vi "Check for Devices Present.vi"(6 "stop notifier reference":refnum<notifier>, 8 "error in":errorcluster, 10 "Devices in":T1[](array[typedef]), 11 "Startup Optimization in":refnum<class "Startup Optimization.lvclass">) -> (0 "error out":errorcluster, 2 "Failed Devices":T1[](array[typedef]), 3 "Startup Optimization out":refnum<class "Startup Optimization.lvclass">, 4 "Time has Elapsed":bool)   [LabVIEW 2018, in "Startup Optimization Actor.lvlib" / "Startup Optimization.lvclass"]
doc: "Ensure all devices that have been told to activate have been activated."
uses:
  Startup Optimization.lvclass
  <vilib>/ORNL/CSEISMIC DDS/CSEISMIC DDS Base/Data Types/Controls/DeviceID.ctl
  C:/Users/Administrator/Desktop/2018LabVIEW EMS/EMS Generic Actor/EMS Generic/EMS Generic.lvclass
  EMS Generic Actor/EMS Generic/EMS Generic.lvclass
  <vilib>/ORNL/CSEISMIC DDS/CSEISMIC DDS Base/CSEISMIC DDS.lvclass
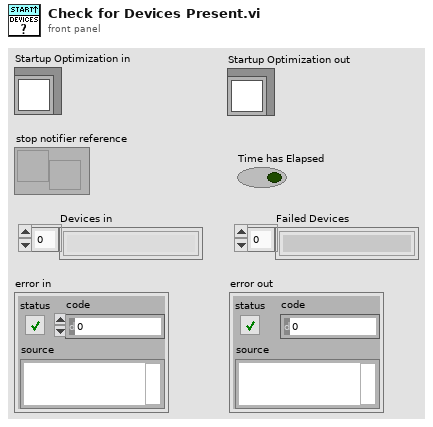
[diagram p1: front panel]
types:
  T1 = typedef "CSEISMIC DDS.lvlib/CSEISMIC DDS.lvclass/DeviceID.ctl" = string
  T2 = typedef "CSEISMIC DDS.lvlib/CSEISMIC DDS.lvclass/IED_Status.ctl" = cluster{"DeviceID":T1, "Timestamp":T3, "MicrogridID":u8, "Active":bool, "Inactive":bool, "Error":i32, "Fault":bool, "ErrorString":string}
  T3 = typedef "CSEISMIC DDS.lvlib/CSEISMIC DDS.lvclass/Timestamp.ctl" = cluster{"Seconds":u64, "Remainder":u64}
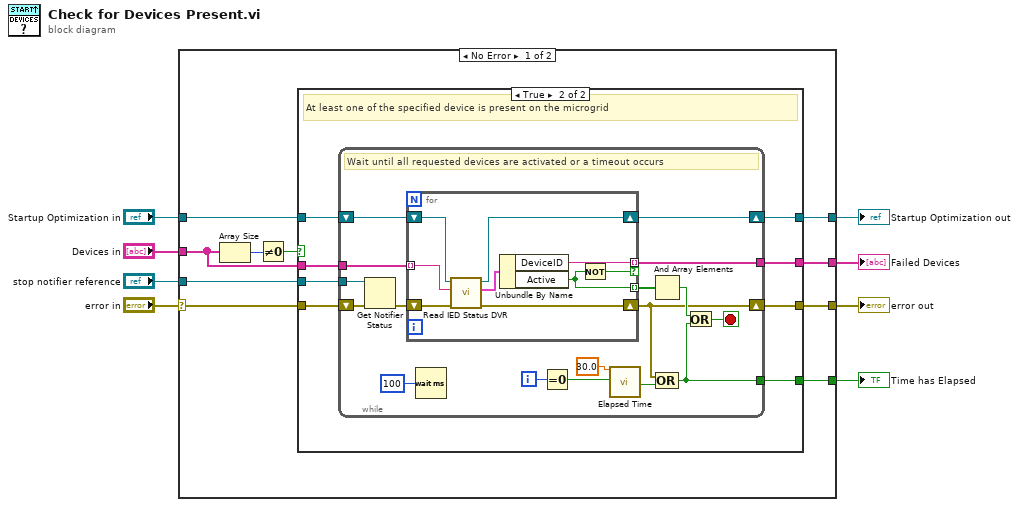
[diagram p0: block diagram]
diagram:
  n1 = case shown="No Error" "error in" {
    selector: "error in" -> [w14 w57]
    tunnel: [w18 w57] -> w8
    tunnel: [w17 w56] -> w7
    tunnel: "stop notifier reference" -> [w16 _]
    tunnel: [w15 _] -> w5
    tunnel: [w11 w55] -> w3
    tunnel: "Startup Optimization in" -> [w10 w55]
    tunnel: "Devices in" -> [w9 w56]
    frame No Error {
      n2 = Array Size(array=w9) -> (size(s)=w12:i32)
      n3 = Not Equal To 0?(x=w12) -> (x != 0?=w13:bool)
      n4 = case shown="True" w13 {
        tunnel: w10 -> [w19 w28]
        tunnel: w9 -> [_ w27]
        tunnel: w14 -> [w20 w26]
        tunnel: [_ w25] -> w15
        tunnel: w16 -> [_ w24]
        tunnel: [_ w23] -> w17
        tunnel: [w20 w22] -> w18
        tunnel: [w19 w21] -> w11
        frame False {
          # "No devices in the list are on the system.  Move to next type of device."
        }
        frame True {
          # "At least one of the specified device is present on the microgrid"
          n5 = while {
            tunnel: w27 -> [w44]
            tunnel: [w38] -> w25
            tunnel: w24 -> [w37]
            tunnel: [w33] -> w23
            shift-right: [w29] -> w22
            shift-left: w26 -> [w32]
            shift-right: [w31] -> w21
            shift-left: w28 -> [w45]
            i -> [w36]
            stop <- w40 stop-if-true
            # "Wait until all requested devices are activated or a timeout occurs"
            n6 = Get Notifier Status(notifier=w37, error in (no error)=w32) -> (error out=w30:errorcluster)  [unwired: 4 out]
            n7 = for {
              tunnel: w44 -> [w49] mode=indexing
              tunnel: [w53] -> w43 mode=indexing
              tunnel: [w54] -> w33 mode=indexing if=w52
              shift-right: [w50] -> w31
              shift-left: w45 -> [w51]
              shift-right: [w46] -> w29
              shift-left: w30 -> [w47]
              n8 = call "Read IED Status DVR.vi"("error in"=w47, "DeviceID"=w49, "EMS Generic in"=w51) -> ("error out"=w46:errorcluster, "IED_Status"=w48:T2, "EMS Generic out"=w50:refnum<class "Startup Optimization.lvclass">)  [unwired: 5 in, 1 out]
              n9 = Unbundle By Name(w48) -> ("DeviceID"=w54:T1, "Active"=w53:bool)
              n10 = Not(x=w53) -> (.not. x?=w52:bool)
            }
            n11 = Wait (ms)(milliseconds to wait=u32 100) -> ()  [unwired: 1 out]
            n12 = Equal To 0?(x=w36) -> (x = 0?=w35:bool)
            n13 = call "Elapsed Time"("Time Target (s)"=30.0, "Reset"=w35) -> ("Time has Elapsed"=w39:bool)  [unwired: 10 in, 7 out]
            n14 = And Array Elements(Boolean array=w43) -> (logical AND=w41:bool)
            n15 = Compound Arithmetic op=OR(w29, w39) -> (w38:bool)
            n16 = Or(x=w41, y=w38) -> (x .or. y?=w40:bool)
          }
        }
      }
    }
    frame Error {
    }
  }
  "error out" <- w8
  "Failed Devices" <- w7
  "Time has Elapsed" <- w5
  "Startup Optimization out" <- w3
